vi "test.write_waveform.vi"   [LabVIEW 2020]
uses:
  Nominal Client/Nominal Client.lvclass
  907d59c3-9021-4a22-baaf-b4b6edfb4b19.vi
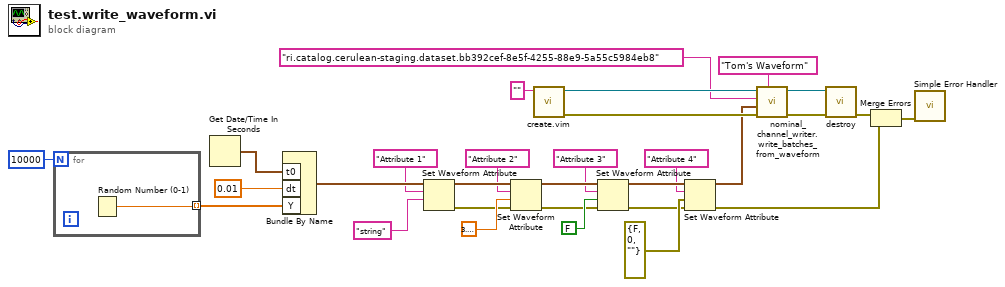
[diagram p0: block diagram]
diagram:
  n1 = for {
    N: 10000 -> [_]
    tunnel: [w31] -> w29 mode=indexing
    n2 = Random Number (0-1)() -> (number: 0 to 1=w31:dbl)
  }
  n3 = Get Date/Time In Seconds() -> (seconds since 1Jan1904=w28:timestamp)
  n4 = Bundle By Name("t0"=w28, "dt"=0.01, "Y"=w29) -> (w26:waveform(dbl))  [unwired: 1 in]
  n5 = Set Waveform Attribute(5:"string" ("name"), 6:"Attribute 1" ("name"), 7:w26) -> (0:w4:errorcluster, 3:w24:waveform(dbl))  [unwired: 1 in, 1 out]
  n6 = Set Waveform Attribute(4:w4, 5:3.141592653589793, 6:"Attribute 2" ("name"), 7:w24) -> (0:w5:errorcluster, 3:w25:waveform(dbl))  [unwired: 1 out]
  n7 = call "create.vim"("API Token (string or path)"="") -> ("error out"=w10:errorcluster, "Nominal Client"=w13:refnum<class "Nominal Client.lvclass">)  [unwired: 9 in]
  n8 = Set Waveform Attribute(4:w5, 5:FALSE, 6:"Attribute 3" ("name"), 7:w25) -> (0:w6:errorcluster, 3:w17:waveform(dbl))  [unwired: 1 out]
  n9 = Set Waveform Attribute(4:w6, 5:errorcluster {"status"=FALSE, "code"=0, "source"=""} ("error in"), 6:"Attribute 4" ("name"), 7:w17) -> (0:w2:errorcluster, 3:w8:waveform(dbl))  [unwired: 1 out]
  n10 = call "nominal_channel_writer.write_batches_from_waveform.vi"("Channel"="Tom's Waveform", "error in"=w10, "Waveform"=w8, "Data Source RID"="ri.catalog.cerulean-staging.dataset.bb392cef-8e5f-4255-88e9-5a55c5984eb8", "Nominal Client in"=w13) -> ("error out"=w11:errorcluster, "Nominal Client out"=w12:refnum<class "Nominal Client.lvclass">)  [unwired: 5 in]
  n11 = call "destroy.vi"("error in"=w11, "Nominal Client"=w12) -> ("error out"=w3:errorcluster)  [unwired: 9 in]
  n12 = Merge Errors(w3, w2) -> (w1:errorcluster)
  n13 = call <vilib>:"Simple Error Handler.vi"("error in (no error)"=w1) -> ()  [unwired: 4 in, 5 out]
